vi "Comm_Initialize(SubVI).vi"(8 "error in (no error)":errorcluster) -> (0 "error out":errorcluster)   [LabVIEW 2017, in "MainFrameLib.lvlib"]
uses:
  MainFrameLib.lvlib
  TypeDefs/FGV_Enum.ctl
  TypeDefs/Command_Enum.ctl
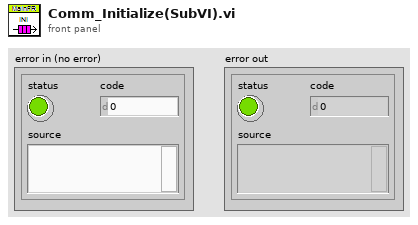
[diagram p1: front panel]
types:
  T1 = typedef "MainFrameLib.lvlib/Command_Enum.ctl" = enum16{"CheckSRLinks", "UpdateKCSColorCode", "StartLinkageCheck", "GetSRNotes", "DisplayAEStats", "InWork&Neglected", "RemapAENames", "ClearFolder", "UpdateReportsList", "ExcelReports", "TeamStats", "LoadReport", "WaitOnReport", "RequestReport", "Error", "Idle", "InitializeData", "ScreenPop", "Initialize", "UpdateCiscoAgentsView", "CancelRequests", "ClipboardCopy", "SaveNeglectedToFile", "Shutdown"}
  T2 = typedef "MainFrameLib.lvlib/FGV_Enum.ctl" = enum16{"Close", "GetRefs", "Initialize"}
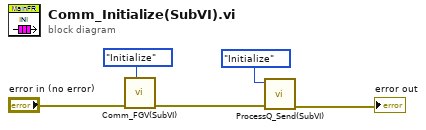
[diagram p0: block diagram]
diagram:
  n1 = call "Comm_FGV(SubVI).vi"("Enum"=FGV_Enum."Initialize", "error in (no error)"="error in (no error)") -> ("error out"=w3:errorcluster)  [unwired: 8 in, 1 out]
  n2 = call "ProcessQ_Send(SubVI).vi"("error in (no error)"=w3, "Command"=Command_Enum."Initialize") -> ("error out"=→"error out":errorcluster)  [unwired: 9 in]
